vi "rhominusdot_decay.vi"(9 "rho- in":dbl[](array[numeric]), 10 "rho0 in":dbl[](array[numeric]), 11 "rho+ in":dbl[](array[numeric])) -> (3 "rho+ dot out":dbl[](array[numeric]))   [LabVIEW 2018]
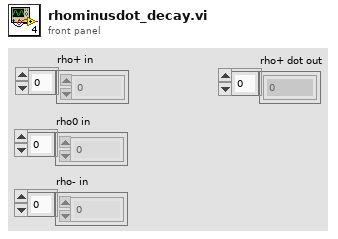
[diagram p1: front panel]
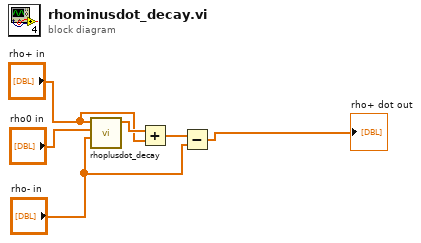
[diagram p0: block diagram]
diagram:
  n1 = call "rhoplusdot_decay.vi"("rho- in"="rho- in", "rho0 in"="rho0 in", "rho+ in"="rho+ in") -> ("rho+ dot out"=w5:dbl[])  [unwired: 8 in]
  n2 = Add(x=w5, y="rho+ in") -> (x+y=w4:dbl[])
  n3 = Subtract(x=w4, y="rho- in") -> (x-y=→"rho+ dot out":dbl[])
